vi "Get Parameter.vi"(8 "error in (no error)":errorcluster, 10 "Parameter":T1, 11 "Sensor General Class in":refnum<class "Sensor General Class.lvclass">) -> (0 "error out":errorcluster, 2 "Data":u16[](array[numeric]), 3 "Sensor General Class out":refnum<class "Sensor General Class.lvclass">)   [LabVIEW 2020, in "Sensor General Class.lvclass"]
uses:
  Sensor General Class.lvclass
  Parameters Enum.ctl
  Sensor General Class.lvclass/Sensor General Class.ctl
  <vilib>/NI Modbus.llb/MB Serial Master Query Read Holding Registers (poly).vi
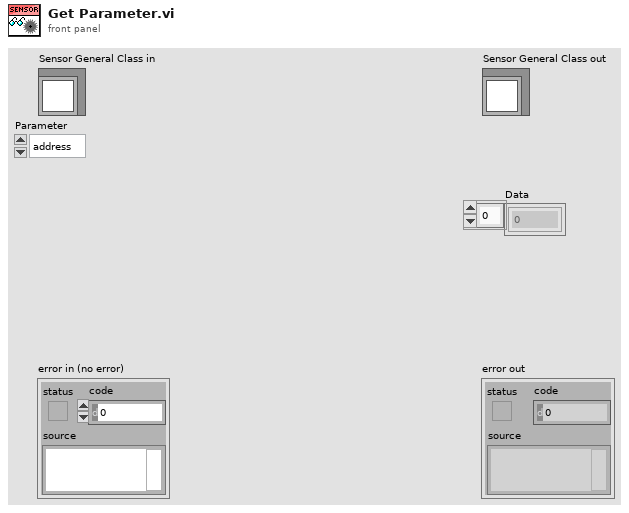
[diagram p1: front panel]
types:
  T1 = typedef "Sensor General Class.lvclass/Parameters Enum.ctl" = enum16{"address", "baud rate", "parity check", "load", "insulating gas", "additional component", "s/n", "hardware version", "firmware version", "humidity enable", "tag", "pressure offset", "humidity offset", "temperature offset", "service code"}
  T2 = cluster{"Mode":enum16{"RTU", "ASCII"}, "Slave Address":u8}
  T3 = cluster{"index":i32, "name":string, "register":u16, "word count":u16, "Write":bool}[]
  T4 = cluster{"index":i32, "name":string, "register":u16, "word count":u16, "Write":bool}
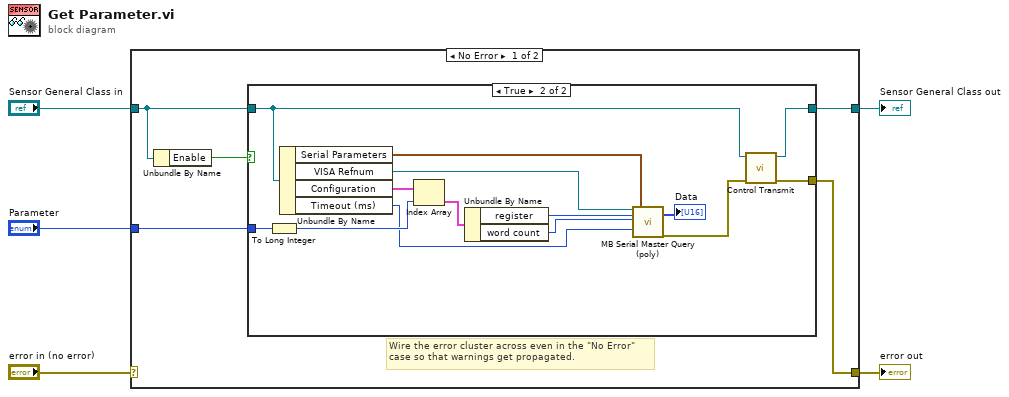
[diagram p0: block diagram]
diagram:
  n1 = case shown="No Error" "error in (no error)" {
    selector: "error in (no error)" -> [_ w27]
    tunnel: [w9 w27] -> w4
    tunnel: [w8 w26] -> w2
    tunnel: "Sensor General Class in" -> [w7 w26]
    tunnel: "Parameter" -> [w10 _]
    frame No Error {
      # "Wire the error cluster across even in the \"No Error\"\ncase so that warnings get propagated."
      n2 = Unbundle By Name(w7) -> ("Enable"=w6:bool)
      n3 = case shown="True" w6 {
        tunnel: w10 -> [_ w16]
        tunnel: w7 -> [w11 w15]
        tunnel: [_ w13] -> w9
        tunnel: [w11 w12] -> w8
        frame False {
        }
        frame True {
          n4 = To Long Integer(number=w16) -> (32bit integer=w22:i32)
          n5 = Unbundle By Name(w15) -> ("Serial Parameters"=w25:T2, "VISA Refnum"=w24:refnum<visa-resource-name>, "Configuration"=w23:T3, "Timeout (ms)"=w19:u32)
          n6 = Index Array(array=w23, index=w22) -> (element=w21:T4)
          n7 = Unbundle By Name(w21) -> ("register"=w20:u16, "word count"=w18:u16)
          n8 = call-poly <vilib>:"MB Serial Master Query (poly).vi"("VISA resource name"=w24, "Starting Address"=w20, "Quantity"=w18, "Timeout"=w19, "Serial Parameters"=w25) -> ("Holding Registers"=→"Data":u16[], "error out"=w14:errorcluster)  [unwired: 11 in, 2 out]
          n9 = call-dynamic "Control Transmit.vi"("error in (no error)"=w14, "Sensor General Class in"=w15) -> ("error out"=w13:errorcluster, "Sensor General Class out"=w12:refnum<class "Sensor General Class.lvclass">)  [unwired: 8 in]
        }
      }
    }
    frame Error {
    }
  }
  "error out" <- w4
  "Sensor General Class out" <- w2
